vi "SimulateJointAngles.vi"() -> ()   [LabVIEW 2016]
panel:
  in  "Stop Button":bool
  in  "q4":dbl(slide) scale=-90.0..90.0
  in  "q3":dbl(slide) scale=-90.0..90.0
  in  "q2":dbl(slide) scale=-90.0..90.0
  in  "q1":dbl(slide) scale=-90.0..90.0
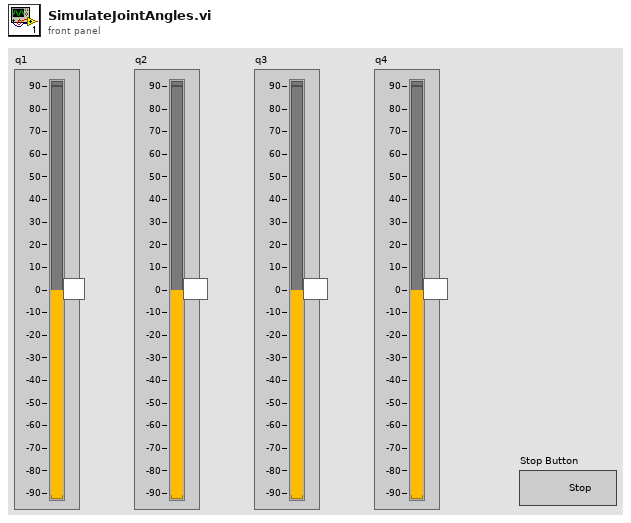
[diagram p1: front panel]
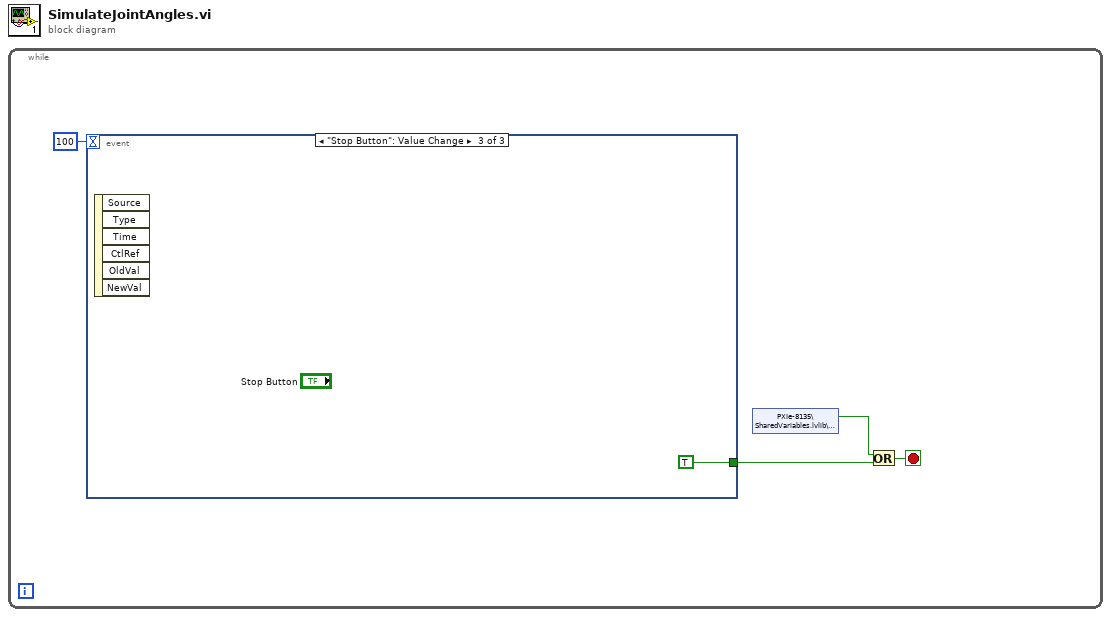
[diagram p0: block diagram]
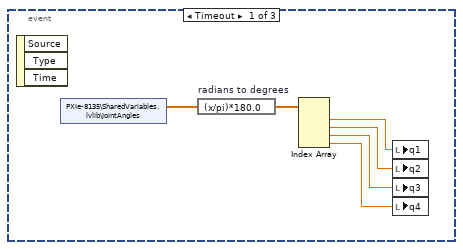
[diagram p2: hidden frame]
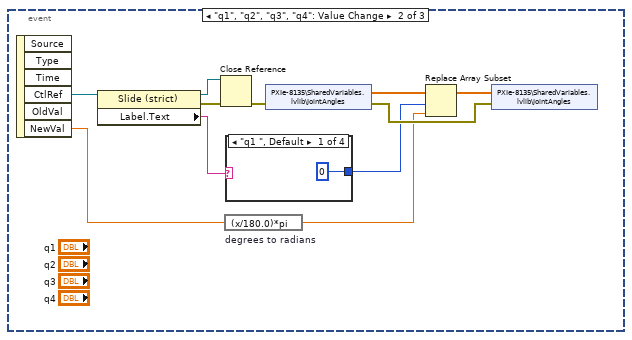
[diagram p3: hidden frame]
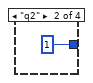
[diagram p4: hidden frame]
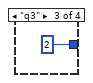
[diagram p5: hidden frame]
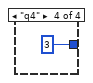
[diagram p6: hidden frame]
diagram:
  n1 = while {
    stop <- w2 stop-if-true
    n2 = event shown="[2] \"Stop Button\": Value Change" {
      selector: _ -> [_ _ _]
      dyn-events: _ -> [_ _ _]
      timeout: 100 -> [_ _ _]
      tunnel: [_ _ TRUE] -> w3
      event Timeout {
        n3 = event-data() -> ()  [unwired: 1 in, 3 out]
        n4 = shared-variable "PXIe-8135\\SharedVariables.lvlib\\JointAngles"() -> (w10:dbl[])  [unwired: 1 in, 1 out]
        n5 = expression code="(x/pi)*180.0" "radians to degrees"(w10) -> (w9:dbl[])
        n6 = Index Array(array=w9) -> (element #1=w8:dbl, element #2=w7:dbl, element #3=w6:dbl, element #4=w5:dbl)  [unwired: 4 in]
        n7 = local write "q1"(w8) -> ()
        n8 = local write "q2"(w7) -> ()
        n9 = local write "q3"(w6) -> ()
        n10 = local write "q4"(w5) -> ()
      }
      event "q1", "q2", "q3", "q4": Value Change {
        n11 = event-data() -> ("CtlRef"=w18:refnum<vi>, "NewVal"=w12:dbl)  [unwired: 1 in, 4 out]
        n12 = property class="Slide (strict)"(reference=w18) -> (reference out=w15:refnum<vi>, error out=w16:errorcluster, "Label.Text"=w17:string)  [unwired: 1 in]
        n13 = Close Reference(reference=w15, error in (no error)=w16) -> (error out=w14:errorcluster)
        n14 = expression code="(x/180.0)*pi" "degrees to radians"(w12) -> (w11:dbl)
        n15 = case shown="\"q1 \", Default" w17 {
          tunnel: [0 1 2 3] -> w13
          frame "q1 ", Default {
          }
          frame "q2" {
          }
          frame "q3" {
          }
          frame "q4" {
          }
        }
        n16 = shared-variable "PXIe-8135\\SharedVariables.lvlib\\JointAngles"(error in=w14) -> (w21:dbl[], error out=w19:errorcluster)
        n17 = Replace Array Subset(array=w21, new element=w11, index=w13) -> (w20:dbl[])
        n18 = shared-variable "PXIe-8135\\SharedVariables.lvlib\\JointAngles"(w20, error in=w19) -> ()  [unwired: 1 out]
      }
      event "Stop Button": Value Change {
        n19 = event-data() -> ()  [unwired: 1 in, 6 out]
      }
    }
    n20 = shared-variable "PXIe-8135\\SharedVariables.lvlib\\Stop RT"() -> (w1:bool)  [unwired: 1 in, 1 out]
    n21 = Or(x=w1, y=w3) -> (x .or. y?=w2:bool)
  }
